vi "차트이미지(subVI).vi"(8 "에러 입력(에러 없음)":errorcluster, 10 "경로":path, 11 "WaveformChart 입력":refnum<vi>) -> ()   [LabVIEW 2014]
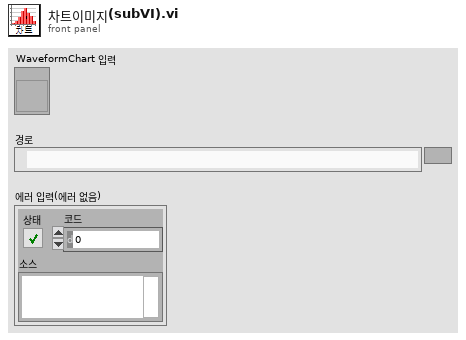
[diagram p1: front panel]
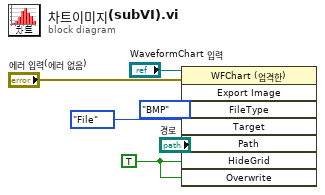
[diagram p0: block diagram]
diagram:
  w5 = TRUE ("눈금 숨기기")
  n1 = invoke on="인보크 노드" class="WFChart (엄격한)" method="Export Image"(reference="WaveformChart 입력", error in="에러 입력(에러 없음)", "FileType"=enum32{"BMP", "EPS", "EMF", "PICT"}."BMP" ("파일 타입"), "Target"=enum32{"File", "Clipboard"}."File" ("타겟"), "Path"="경로", "HideGrid"=w5, "Overwrite"=w5) -> ()  [unwired: 1 in, 8 out]
